vi "AcquireHardware.vi"(8 "error in (no error)":errorcluster, 11 "SkySparkDevice in":refnum<class "SkySparkDevice.lvclass">) -> (0 "error out":errorcluster, 3 "SkySparkDevice out":refnum<class "SkySparkDevice.lvclass">)   [LabVIEW 2020, in "SkySparkDevice.lvclass"]
uses:
  SkySparkDevice.lvclass
  FGVFunctionTypeDef.ctl
  FGV_TypeDef.ctl
  SkySparkDevice.lvclass/SkySparkDevice.ctl
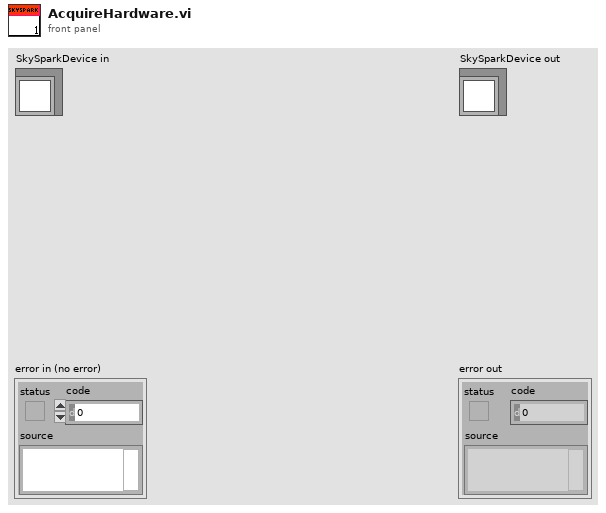
[diagram p1: front panel]
types:
  T1 = typedef "SkySparkDevice.lvclass/FGV_TypeDef.ctl" = cluster{"Data_Array":string[][], "Busy":bool}
  T2 = typedef "SkySparkDevice.lvclass/FGVFunctionTypeDef.ctl" = enum16{"Clear", "Write", "Read"}
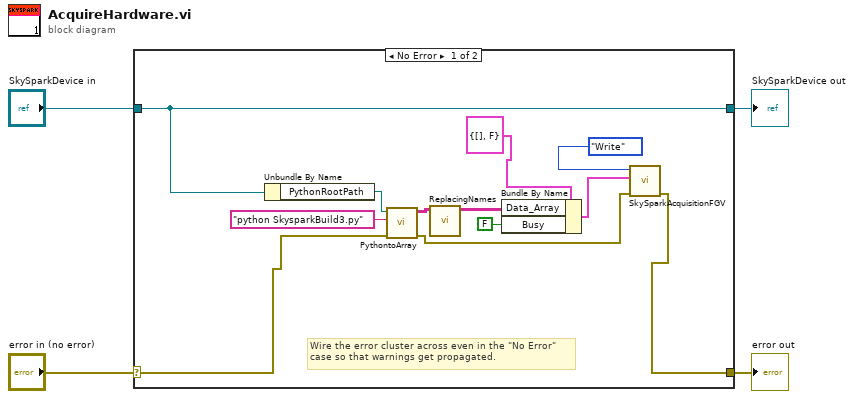
[diagram p0: block diagram]
diagram:
  n1 = case shown="No Error" "error in (no error)" {
    selector: "error in (no error)" -> [w12 w18]
    tunnel: [w6 w18] -> w3
    tunnel: [w13 w17] -> w1
    tunnel: "SkySparkDevice in" -> [w13 w17]
    frame No Error {
      # "Wire the error cluster across even in the \"No Error\"\ncase so that warnings get propagated."
      n2 = Unbundle By Name(w13) -> ("PythonRootPath"=w15:path)
      n3 = call "PythontoArray.vi"("error in (no error)"=w12, "command line"="python SkysparkBuild3.py", "working directory"=w15) -> ("error out"=w7:errorcluster, "Output Array"=w14:string[][])  [unwired: 6 in, 1 out]
      n4 = call "ReplacingNames.vi"("Input Array"=w14) -> ("output array"=w9:string[][])  [unwired: 10 in]
      n5 = Bundle By Name(cluster=T1 {"Data_Array"=[], "Busy"=FALSE} ("FGV_Cluster"), "Data_Array"=w9, "Busy"=FALSE) -> (w8:T1)
      n6 = call "SkySparkAcquisitionFGV.vi"("error in (no error)"=w7, "FGV_Cluster Input"=w8, "Function"=FGVFunctionTypeDef."Write") -> ("error out"=w6:errorcluster)  [unwired: 7 in, 1 out]
    }
    frame Error {
    }
  }
  "error out" <- w3
  "SkySparkDevice out" <- w1
